vi "Symphony Format AreaV2.vi"(4 "Y Start":i32=255 min=1 max=255 step=1, 5 "Y End":i32=256 min=1 max=256 step=1, 6 "ImageMode":bool, 7 "error in (no error)":errorcluster, 8 "X Start":i32=1023 min=1 max=1023 step=1, 9 "X End":i32=1024 min=1 max=1024 step=1, 10 "numAreas":i32=1) -> (0 "error out":errorcluster, 2 "areas :":i32[][](array[numeric])=[[1], [1], [1], [1024], [256], [1], [256]], 3 "X Size Out":i32=1024 min=1 max=1024 step=1)   [LabVIEW 2012]
panel:
  # "Area#"
  # "X Origin"
  # "Y Origin"
  # "X Size"
  # "Y Size"
  # "X Bin"
  # "Y Bin"
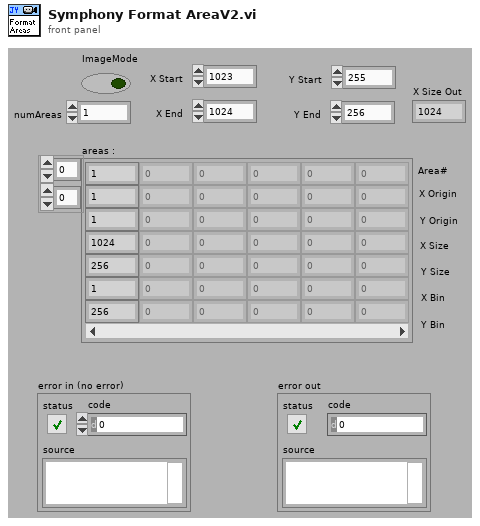
[diagram p1: front panel]
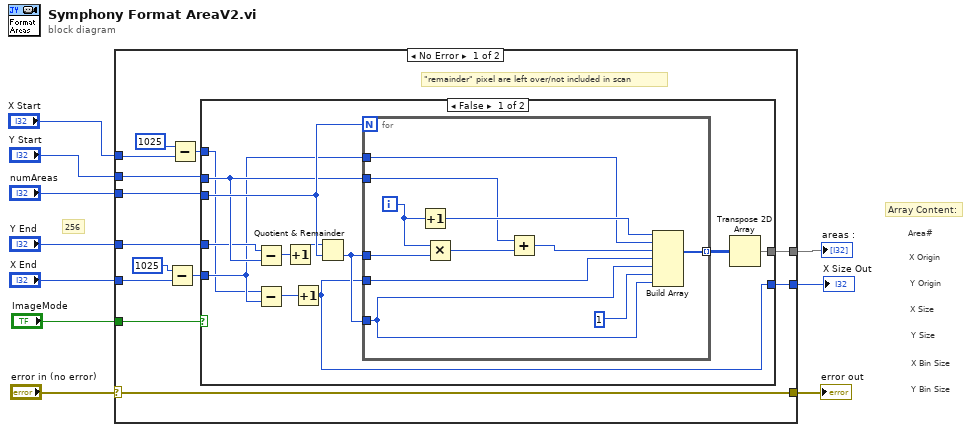
[diagram p0: block diagram]
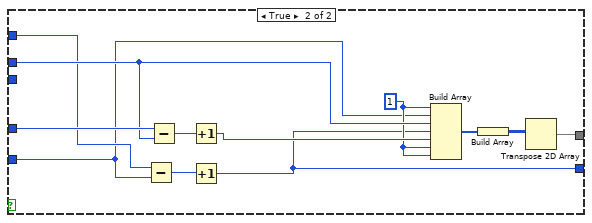
[diagram p2: hidden frame]
diagram:
  # "256"
  # "Array Content:"
  # "Y Bin Size"
  # "X Bin Size"
  # "Y Size"
  # "X Size"
  # "Y Origin"
  # "X Origin"
  # "Area#"
  n1 = case shown="No Error" "error in (no error)" {
    selector: "error in (no error)" -> [w21 w59]
    tunnel: "numAreas" -> [w23 _]
    tunnel: [w22 _] -> w9
    tunnel: "X End" -> [w11 _]
    tunnel: "Y End" -> [w19 _]
    tunnel: [w21 w59] -> w5
    tunnel: "X Start" -> [w14 _]
    tunnel: "Y Start" -> [w20 _]
    tunnel: "ImageMode" -> [w18 _]
    tunnel: [w17 _] -> w1
    frame No Error {
      # "\"remainder\" pixel are left over/not included in scan"
      n2 = Subtract(x=1025, y=w11) -> (x-y=w12:i32)
      n3 = Subtract(x=1025, y=w14) -> (x-y=w15:i32)
      n4 = case shown="False" w18 {
        tunnel: w23 -> [w35 _]
        tunnel: [w33 w50] -> w22
        tunnel: w20 -> [w31 w55]
        tunnel: w19 -> [w30 w57]
        tunnel: w12 -> [w25 w47]
        tunnel: w15 -> [w24 w48]
        tunnel: [w26 w49] -> w17
        frame False {
          n5 = Subtract(x=w30, y=w31) -> (x-y=w28:i32)
          n6 = Subtract(x=w24, y=w25) -> (x-y=w27:i32)
          n7 = Increment(x=w28) -> (x+1=w29:i32)
          n8 = Increment(x=w27) -> (x+1=w26:i32)
          n9 = Quotient & Remainder(x=w29, y=w35) -> (floor(x/y)=w32:i32)  [unwired: 1 out]
          n10 = for {
            N: w35 -> [_]
            tunnel: w32 -> [w44]
            tunnel: [w46] -> w34 mode=indexing
            tunnel: w32 -> [w41]
            tunnel: w26 -> [w40]
            tunnel: w25 -> [w39]
            tunnel: w31 -> [w37]
            i -> [w43]
            n11 = Increment(x=w43) -> (x+1=w42:i32)
            n12 = Multiply(x=w43, y=w44) -> (x*y=w36:i32)
            n13 = Add(x=w37, y=w36) -> (x+y=w38:i32)
            n14 = Build Array(w42, w39, w38, w40, w41, 1, w41) -> (w46:i32[])
          }
          n15 = Transpose 2D Array(2D array=w34) -> (transposed array=w33:i32[][])
        }
        frame True {
          w52 = 1 ("numAreas")
          n16 = Subtract(x=w48, y=w47) -> (x-y=w53:i32)
          n17 = Subtract(x=w57, y=w55) -> (x-y=w56:i32)
          n18 = Increment(x=w56) -> (x+1=w54:i32)
          n19 = Increment(x=w53) -> (x+1=w49:i32)
          n20 = Build Array(w52, w47, w55, w49, w54, w52, w52) -> (w58:i32[])
          n21 = Build Array(w58) -> (w51:i32[][])
          n22 = Transpose 2D Array(2D array=w51) -> (transposed array=w50:i32[][])
        }
      }
    }
    frame Error {
    }
  }
  "error out" <- w5
  "areas :" <- w9
  "X Size Out" <- w1
